vi "Go To Angle.vi"(6 "wait for reply (T)":bool=TRUE, 7 "Pause Time [ms]":i32=50, 8 "error in":errorcluster, 9 "Velocity [rpm]":i32=5, 10 "Angle":dbl, 11 "Module ID":i32=-1) -> (0 "error out":errorcluster, 1 "timed out?":bool, 2 "Angle 2":dbl)   [LabVIEW 2025, in "Stepper.lvlib"]
doc: "_____\nCreated using DQMH Framework: Event Scripter 7.1.2.1547."
uses:
  Stepper.lvlib
  Go To Angle Argument--cluster.ctl
  Go To Angle (Reply Payload)--cluster.ctl
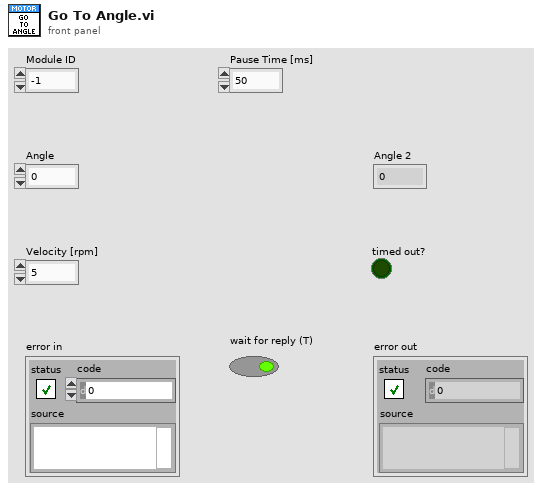
[diagram p1: front panel]
types:
  T1 = typedef "Stepper.lvlib/Go To Angle Argument--cluster.ctl" = cluster{"Module ID":i32, "Angle":dbl, "Velocity [rpm]":i32, "Pause Time [ms]":i32, "Wait Notifier":refnum<notifier>, "wait for reply":bool}
  T2 = typedef "Stepper.lvlib/Request Events--cluster.ctl" = cluster{"Stop Module":refnum<user-event>, "Show Panel":refnum<user-event>, "Hide Panel":refnum<user-event>, "Show Diagram":refnum<user-event>, "Get Module Execution Status":refnum<user-event>, "close":refnum<user-event>, "init":refnum<user-event>, "init driver":refnum<user-event>, "Clear Motor Error":refnum<user-event>, "read config":refnum<user-event>, "Read Angle":refnum<user-event>, "Jog":refnum<user-event>, "Go To Angle":refnum<user-event>}
  T3 = typedef "Stepper.lvlib/Go To Angle (Reply Payload)--cluster.ctl" = cluster{"Module ID":i32, "Angle":dbl, "error":errorcluster}
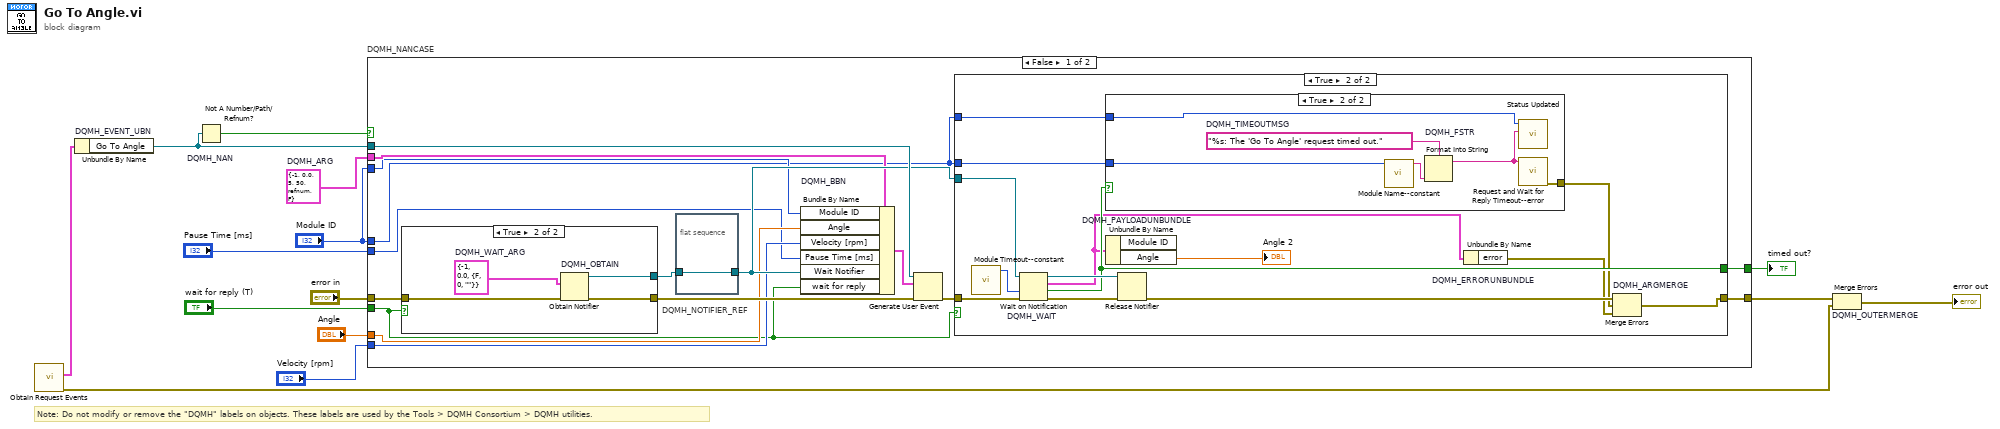
[diagram p0: block diagram]
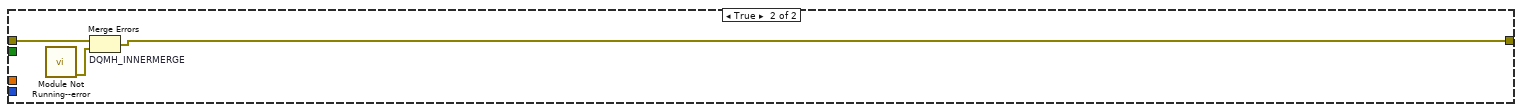
[diagram p5: hidden frame]
diagram:
  w8 = T1 {"Module ID"=-1, "Angle"=0.0, "Velocity [rpm]"=5, "Pause Time [ms]"=50, "Wait Notifier"=refnum, "wait for reply"=FALSE}  # DQMH_ARG
  # "Note: Do not modify or remove the \"DQMH\" labels on objects. These labels are used by the Tools > DQMH Consortium > DQMH utilities."
  n1 = call "Obtain Request Events.vi"() -> ("error out"=w2:errorcluster, "Stepper Request Events"=w1:T2)  [unwired: 10 in]
  n2 = Unbundle By Name "DQMH_EVENT_UBN"(w1) -> ("Go To Angle"=w12:refnum<user-event>)
  n3 = Not A Number/Path/Refnum? "DQMH_NAN"(number/path/refnum=w12) -> (NaN/Path/Refnum?=w11:bool)
  n4 = case "DQMH_NANCASE" shown="False" w11 {
    tunnel: "error in" -> [w30 w60]
    tunnel: w12 -> [w28 _]
    tunnel: [w25 w59] -> w9
    tunnel: [w26 _] -> w10
    tunnel: w8 -> [w21 _]
    tunnel: "Module ID" -> [w20 _]
    tunnel: "Angle" -> [w19 _]
    tunnel: "Velocity [rpm]" -> [w18 _]
    tunnel: "Pause Time [ms]" -> [w17 _]
    tunnel: "Module ID" -> [w16 _]
    tunnel: "wait for reply (T)" -> [w15 _]
    frame False {
      n5 = case shown="True" w15 {
        tunnel: w30 -> [w53 w57]
        tunnel: [w53 w56] -> w27
        tunnel: [_ w54] -> w23
        frame False {
        }
        frame True {
          w55 = T3 {"Module ID"=-1, "Angle"=0.0, "error"={"status"=FALSE, "code"=0, "source"=""}}  # DQMH_WAIT_ARG
          n6 = Obtain Notifier "DQMH_OBTAIN"(notification data type=w55, error in (no error)=w57) -> (notifier out=w54:refnum<notifier>, error out=w56:errorcluster)  [unwired: 2 in, 1 out]
        }
      }
      n7 = flat-sequence "DQMH_NOTIFIER_REF" {
        tunnel: w23 -> [w31]
        tunnel: [w31] -> w22
        frame #0 {
        }
      }
      n8 = Bundle By Name "DQMH_BBN"(cluster=w21, "Module ID"=w20, "Angle"=w19, "Velocity [rpm]"=w18, "Pause Time [ms]"=w17, "Wait Notifier"=w22, "wait for reply"=w15) -> (w24:T1)
      n9 = Generate User Event(user event=w28, event data cluster=w24, error in=w27) -> (error out=w29:errorcluster)  [unwired: 1 in, 1 out]
      n10 = case shown="True" w15 {
        tunnel: w29 -> [w32 w46]
        tunnel: w22 -> [_ w45]
        tunnel: [_ w43] -> w26
        tunnel: [w32 w42] -> w25
        tunnel: w16 -> [_ w34]
        tunnel: w16 -> [_ w33]
        frame False {
        }
        frame True {
          n11 = call "Module Timeout--constant.vi"() -> ("Module Timeout"=w36:i32)  [unwired: 11 in]
          n12 = Wait on Notification "DQMH_WAIT"(notifier=w45, timeout in ms (-1)=w36, error in (no error)=w46) -> (notifier out=w44:refnum<notifier>, notification=w37:T3, timed out?=w43:bool, error out=w41:errorcluster)  [unwired: 1 in]
          n13 = case shown="True" w43 {
            tunnel: [_ w50] -> w38
            tunnel: w34 -> [_ w48]
            tunnel: w33 -> [_ w47]
            frame False {
            }
            frame True {
              w52 = "%s: The 'Go To Angle' request timed out."  # DQMH_TIMEOUTMSG
              n14 = call "Module Name--constant.vi"("Module ID"=w47) -> ("Module Name"=w49:string)  [unwired: 10 in]
              n15 = Format Into String "DQMH_FSTR"(format string=w52, w49) -> (resulting string=w51:string)  [unwired: 2 in, 1 out]
              n16 = call "Status Updated.vi"("Status"=w51, "Module ID"=w48) -> ()  [unwired: 9 in, 1 out]
              n17 = call "Request and Wait for Reply Timeout--error.vi"("Error Message"=w51) -> ("error out"=w50:errorcluster)  [unwired: 10 in]
            }
          }
          n18 = Unbundle By Name "DQMH_PAYLOADUNBUNDLE"(w37) -> ("Angle"=→"Angle 2":dbl)  [unwired: 1 out]
          n19 = Release Notifier(notifier=w44, error in (no error)=w41) -> (error out=w40:errorcluster)  [unwired: 1 in, 2 out]
          n20 = Unbundle By Name "DQMH_ERRORUNBUNDLE"(w37) -> ("error"=w39:errorcluster)
          n21 = Merge Errors "DQMH_ARGMERGE"(w40, w38, w39) -> (w42:errorcluster)
        }
      }
    }
    frame True {
      n22 = call "Module Not Running--error.vi"() -> ("error out"=w58:errorcluster)  [unwired: 11 in]
      n23 = Merge Errors "DQMH_INNERMERGE"(w60, w58) -> (w59:errorcluster)
    }
  }
  "timed out?" <- w10
  n24 = Merge Errors "DQMH_OUTERMERGE"(w9, w2) -> (→"error out":errorcluster)
